vi "Global_FW_RPM_In.vi"() -> ()   [LabVIEW 2017]
panel:
  in  "Fly Wheel RPM Input":dbl
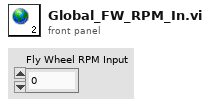
[diagram p1: front panel]
diagram:
